vi "Arcade Drive.vi"(4 "b":dbl=1.0, 5 "a":dbl=1.0, 7 "Metrics In":T1) -> (3 "Metrics Out":T1)   [LabVIEW 2014]
uses:
  Drive Train/Drive Metrics.ctl
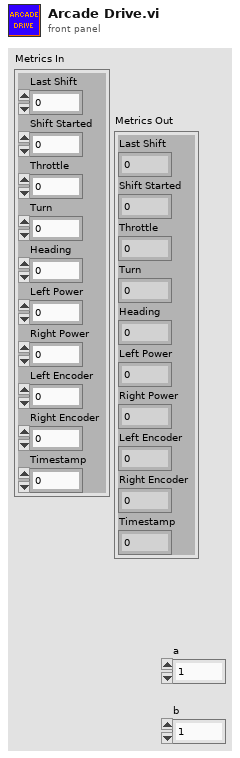
[diagram p1: front panel]
types:
  T1 = typedef "Drive Metrics.ctl" = cluster{"Last Shift":u32, "Shift Started":u32, "Throttle":dbl, "Turn":dbl, "Heading":dbl, "Left Power":dbl, "Right Power":dbl, "Left Encoder":dbl, "Right Encoder":dbl, "Timestamp":dbl}
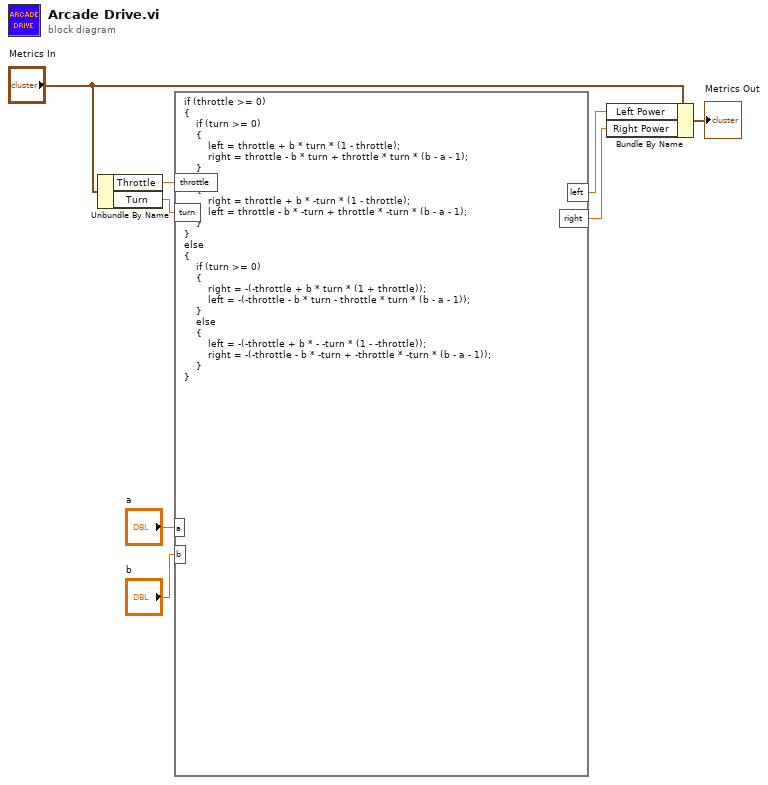
[diagram p0: block diagram]
diagram:
  n1 = Unbundle By Name("Metrics In") -> ("Throttle"=w6:dbl, "Turn"=w5:dbl)
  n2 = formula code="if (throttle >= 0)\n{\n    if (turn >= 0)\n    {\n        left = throttle + b * turn * (1 - throttle);\n        right = throttle - b * turn + throttle * turn * (b - a - 1);\n    }\n    else\n    {\n        right = throttle + b * -turn * (1 - throttle);\n        left = throttle - b * -turn + throttle * -turn * (b - a - 1);\n    }\n}\nelse\n{\n    if (turn >= 0)\n    {\n        right = -(-throttle + b * turn * (1 + throttle));\n        left = -(-throttle - b * turn - throttle * turn * (b - a - 1));\n    }\n    else\n    {\n        left = -(-throttle + b * - -turn * (1 - -throttle));\n        right = -(-throttle - b * -turn + -throttle * -turn * (b - a - 1));\n    }\n}"("throttle"=w6, "turn"=w5, "a"="a", "b"="b") -> ("left"=w2:dbl, "right"=w1:dbl)
  n3 = Bundle By Name(cluster="Metrics In", "Left Power"=w2, "Right Power"=w1) -> (→"Metrics Out":T1)
